vi "未命名 3.vi"(0 "Image In":T3, 1 "Image Dst":T3, 2 "ROI Descriptor (Pattern Matching 1)":T2={"Global Rectangle"=[20, 78, 890, 919], "Contours"=[{"ID"=enum."External", "Type"=12, "Coordinates"=[20, 78, 890, 919, 0]}]} {"Contours"."Type" items=["No Selection", "Point", "Line", "Rectangle", "Oval", "Polygon", "Freehand Region", "Annulus", "Unused2", "Unused3", "Broken Line", "Freehand Line", "Rotated Rectangle"]}, 3 "Algorithm (Pattern Matching 1)":i32(ring)=2 items=["All", "Low Discrepancy Sampling", "Grayscale Value Pyramid", "Gradients Pyramid"], 4 "Parameters (Pattern Matching 1)":T1={"Number of Matches Requested"=1, "Minimum Match Score"=800.0, "Angle Ranges"=[]}, 5 "Advanced Options (Pattern Matching 1)":cluster{"Item":u16, "Value":dbl}[](array[cluster])=[{"Item"=102, "Value"=10.0}, {"Item"=106, "Value"=300.0}, {"Item"=107, "Value"=0.0}, {"Item"=108, "Value"=6.0}, {"Item"=109, "Value"=1.0}, {"Item"=114, "Value"=25.0}, {"Item"=111, "Value"=20.0}, {"Item"=112, "Value"=10.0}, {"Item"=113, "Value"=20.0}, {"Item"=103, "Value"=1.0}, {"Item"=104, "Value"=20.0}, {"Item"=105, "Value"=0.0}, {"Item"=100, "Value"=6.0}] {"Item" items=["LD Sampling - Minimum Constrast"=0, "LD Sampling - Enable Subpixel Accuracy"=1, "LD Sampling - Search Strategy"=2, "LD Sampling - Subpixel Iterations"=3, "LD Sampling - Subpixel Tolerance"=4, "LD Sampling - Initial Match List Length"=5, "LD Sampling - Match List Reduction Factor"=6, "LD Sampling - Initial Step Size"=7, "LD Sampling - Intermediate Angular Accuracy"=8, "-"=9, "Pyramid - Max Pyramid Level"=100, "Pyramid - Minimum Contrast"=102, "Pyramid - Enable Subpixel Accuracy"=103, "Pyramid - Subpixel Iterations"=104, "Pyramid - Subpixel Tolerance"=105, "Pyramid - Initial Match List Length"=106, "Pyramid - Match List Reduction Factor"=107, "Pyramid - Intermediate Angular Accuracy"=108, "Pyramid - Process Border Matches"=109, "Pyramid - Min Match Separation Distance"=111, "Pyramid - Min Match Separation Angle"=112, "Pyramid - Max Match Overlap"=113, "Pyramid - Max Cache in MB"=114, "Pyramid - Clear Cache"=115, "-"=116, "Enable Defect Map"=200]}, 6 "Template File Path (Pattern Matching 1)":path=path "D:/Inspect System/Source Code/Template Program/字符检测定位模板.png", 7 "error in":errorcluster) -> (20 "Image Out":T3, 21 "Matches (Pattern Matching 1)":T4(array[cluster]) {"Bounding Box"."y" format="%.2f"; "Bounding Box"."x" format="%.2f"; "Position"."y" format="%.2f"; "Position"."x" format="%.2f"; "Score" format="%.2f"; "Scale" format="%.2f"; "Angle" format="%.2f"}, 22 "Calibrated Matches (Pattern Matching 1)":T4(array[cluster]) {"Bounding Box"."y" format="%.2f"; "Bounding Box"."x" format="%.2f"; "Position"."y" format="%.2f"; "Position"."x" format="%.2f"; "Score" format="%.2f"; "Scale" format="%.2f"; "Angle" format="%.2f"}, 23 "Number of Matches (Pattern Matching 1)":i32, 27 "error out":errorcluster)   [LabVIEW 2017]
doc: "Creates, edits, and runs vision algorithms using NI Vision Assistant.\n\nWhen you place this Express VI on the block diagram, NI Vision Assistant launches. Create an algorithm using the Vision Assistant processing functions. After you create an algorithm, you can select the controls and indicators that you want to be able to programmatically set in LabVIEW. Double-click the Vision Assistant Express VI to edit the algorithm."
uses:
  <vilib>/vision/Image Controls.llb/IMAQ Image.ctl
  <vilib>/vision/NI_Vision_Development_Module.lvlib
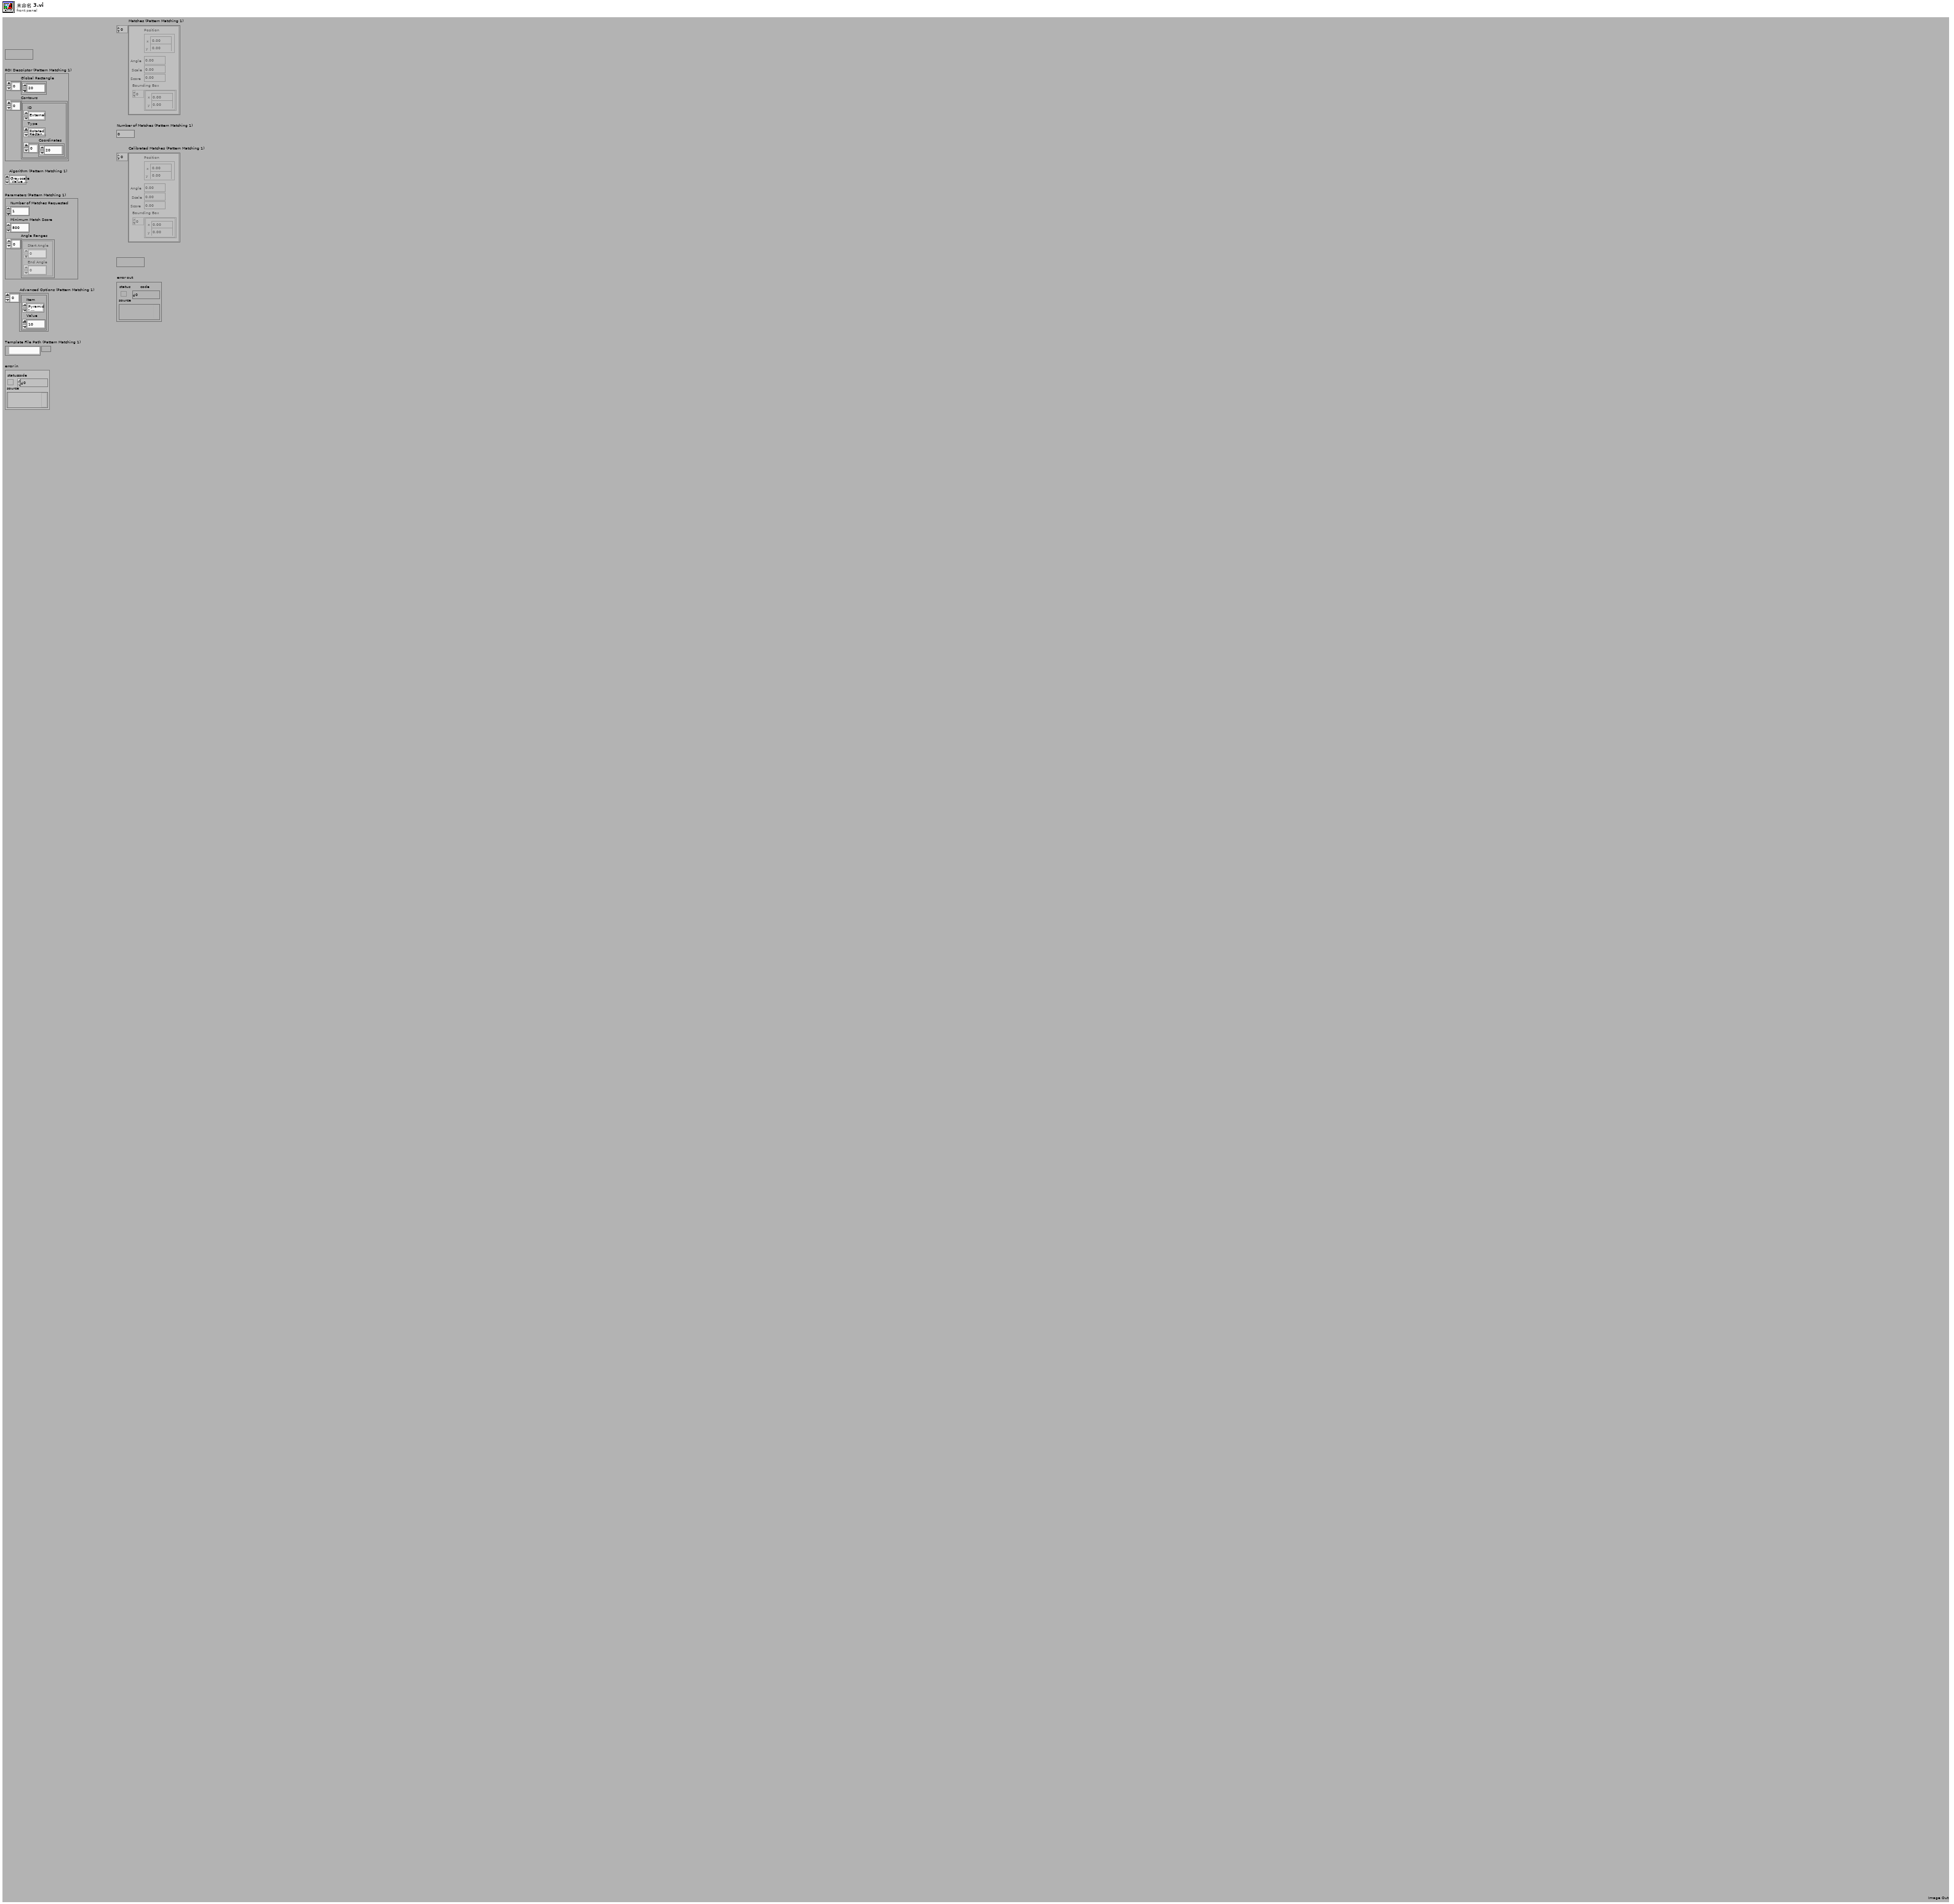
[diagram p1: front panel]
types:
  T1 = cluster{"Number of Matches Requested":i32, "Minimum Match Score":sgl, "Angle Ranges":cluster{"Start Angle":sgl, "End Angle":sgl}[]}
  T2 = cluster{"Global Rectangle":i32[], "Contours":cluster{"ID":enum32{"External", "Internal"}, "Type":u32, "Coordinates":i32[]}[]}
  T3 = typedef "IMAQ Image.ctl" = refnum<image>
  T4 = cluster{"Position":cluster{"x":sgl, "y":sgl}, "Angle":sgl, "Scale":sgl, "Score":sgl, "Bounding Box":cluster{"x":sgl, "y":sgl}[]}[]
  T5 = typedef "Image Type" = u32
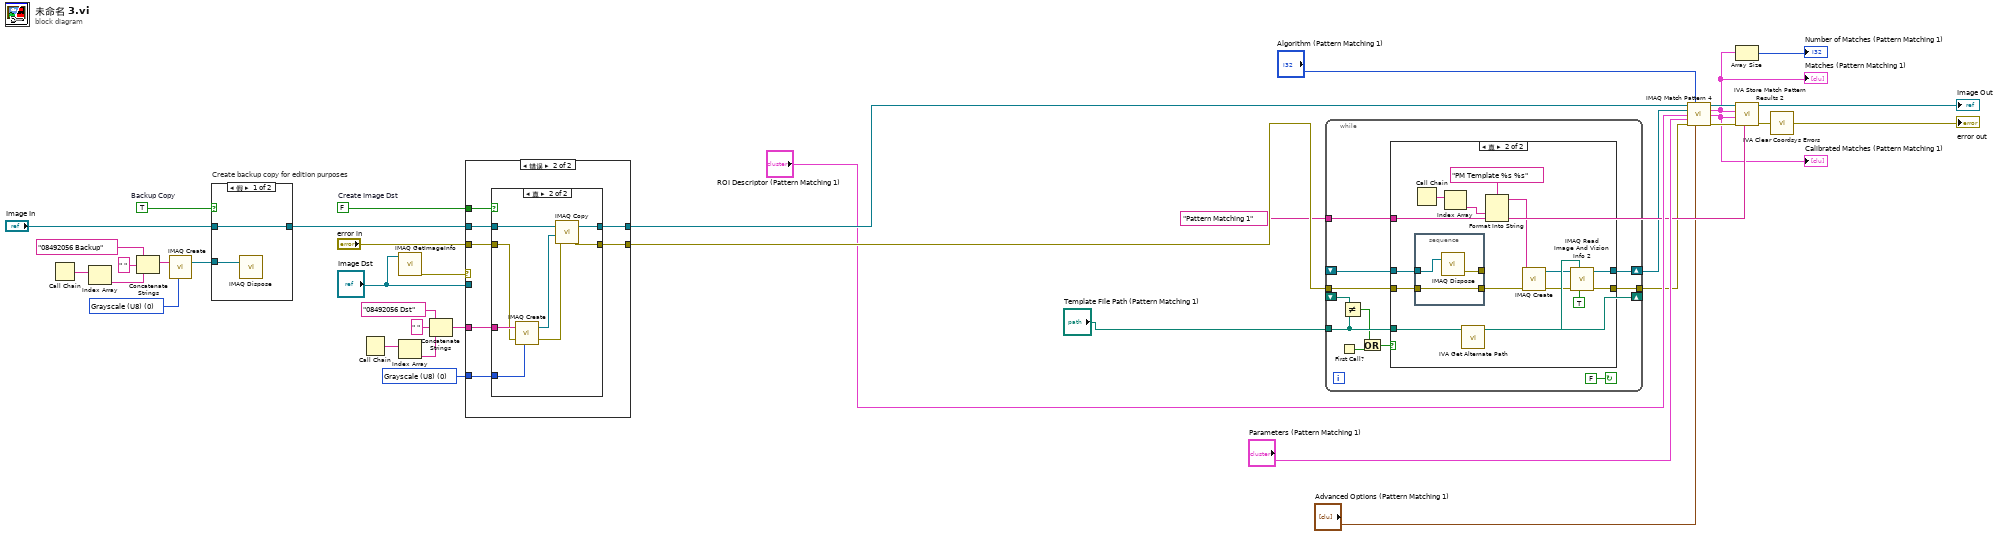
[diagram p0: block diagram]
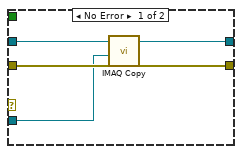
[diagram p3: hidden frame]
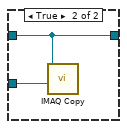
[diagram p5: hidden frame]
diagram:
  w9 = "Pattern Matching 1" ("Step Name")
  w18 = T5 0 items=["Grayscale (U8)", "Grayscale (I16)", "Grayscale (SGL)", "Complex (CSG)", "RGB (U32)", "HSL (U32)", "RGB (U64)", "Grayscale (U16)"] ("Image Dst Type")
  w19 = T5 0 items=["Grayscale (U8)", "Grayscale (I16)", "Grayscale (SGL)", "Complex (CSG)", "RGB (U32)", "HSL (U32)", "RGB (U64)", "Grayscale (U16)"] ("Image Type")
  w38 = TRUE  # Backup Copy
  w31 = FALSE  # Create Image Dst
  n1 = Call Chain() -> (call chain=w25:string[])
  n2 = Index Array(array=w25) -> (element=w24:string)  [unwired: 1 in]
  n3 = Concatenate Strings("08492056 Backup" ("Backup Image Name"), " ", w24) -> (w21:string)
  n4 = call "IMAQ Create"("Image Name"=w21, "Image Type"=w19) -> ("New Image"=w20:T3)  [unwired: 2 in, 2 out]
  n5 = case "Create backup copy for edition purposes" shown="假" w38 {
    tunnel: [w40 w42] -> w34
    tunnel: "Image In" -> [w40 w42]
    tunnel: w20 -> [w39 w41]
    frame False {
      n6 = call "IMAQ Dispose"("Image"=w39) -> ()  [unwired: 2 in, 4 out]
    }
    frame True {
      n7 = call "IMAQ Copy"("Image Dst"=w41, "Image Src"=w42) -> ()  [unwired: 1 in, 5 out]
    }
  }
  n8 = Call Chain() -> (call chain=w30:string[])
  n9 = call "IMAQ GetImageInfo"("Image"="Image Dst") -> ("error out"=w36:errorcluster)  [unwired: 1 in, 9 out]
  n10 = Index Array(array=w30) -> (element=w28:string)  [unwired: 1 in]
  n11 = Concatenate Strings("08492056 Dst" ("Image Dst Name"), " ", w28) -> (w26:string)
  n12 = case "条件结构" shown="错误" w36 {
    tunnel: [w47 w51] -> w16
    tunnel: [w46 w50] -> w32
    tunnel: w34 -> [w45 w52]
    tunnel: "error in" -> [w44 w48]
    tunnel: "Image Dst" -> [w43 _]
    tunnel: w26 -> [_ w54]
    tunnel: w18 -> [_ w53]
    tunnel: w31 -> [_ w49]
    frame No Error {
      n13 = call "IMAQ Copy"("error in (no error)"=w44, "Image Dst"=w43, "Image Src"=w45) -> ("error out"=w46:errorcluster, "Image Dst Out"=w47:T3)  [unwired: 3 out]
    }
    frame Error {
      n14 = case "条件结构" shown="真" w49 {
        tunnel: w54 -> [_ w64]
        tunnel: w53 -> [_ w63]
        tunnel: w52 -> [w56 w61]
        tunnel: [w56 w60] -> w51
        tunnel: [w55 w59] -> w50
        tunnel: w48 -> [w55 w57]
        frame False {
        }
        frame True {
          n15 = call "IMAQ Create"("Image Name"=w64, "Image Type"=w63, "error in (no error)"=w57) -> ("New Image"=w62:T3, "error out"=w58:errorcluster)  [unwired: 1 in, 1 out]
          n16 = call "IMAQ Copy"("error in (no error)"=w58, "Image Dst"=w62, "Image Src"=w61) -> ("error out"=w59:errorcluster, "Image Dst Out"=w60:T3)  [unwired: 3 out]
        }
      }
    }
  }
  n17 = while {
    shift-right: [w75] -> w6
    shift-left: _ -> [w74]
    tunnel: [w72] -> w5
    tunnel: w32 -> [w71]
    tunnel: "Template File Path (Pattern Matching 1)" -> [w68]
    tunnel: w9 -> [w70]
    shift-right: [w68] -> _
    shift-left: _ -> [w69]
    stop <- FALSE continue-if-true
    n18 = First Call?() -> (First Call?: T/F=w67:bool)
    n19 = Not Equal?(x=w69, y=w68) -> (x != y?=w66:bool)
    n20 = Or(x=w66, y=w67) -> (x .or. y?=w65:bool)
    n21 = case "条件结构" shown="真" w65 {
      tunnel: [w77 w82] -> w75
      tunnel: w74 -> [w77 w86]
      tunnel: [w76 w83] -> w72
      tunnel: w71 -> [w76 w85]
      tunnel: w68 -> [_ w87]
      tunnel: w70 -> [_ w88]
      frame False {
      }
      frame True {
        n22 = stacked-sequence "层叠式顺序结构" {
          tunnel: w86 -> [w95]
          tunnel: w85 -> [w94]
          tunnel: [w94] -> w79
          tunnel: [w93] -> _
          frame #0 {
            n23 = call "IMAQ Dispose"("Image"=w95) -> ("error out"=w93:errorcluster)  [unwired: 2 in, 3 out]
          }
        }
        n24 = Call Chain() -> (call chain=w90:string[])
        n25 = Index Array(array=w90) -> (element=w89:string)  [unwired: 1 in]
        n26 = call <vilib>:"IVA Get Alternate Path.vi"("Path In"=w87) -> ("Path Out"=w84:path)  [unwired: 10 out]
        n27 = Format Into String(format string="PM Template %s %s" ("Image Name"), w89, w88) -> (resulting string=w92:string)  [unwired: 2 in, 1 out]
        n28 = call "IMAQ Create"("Image Name"=w92, "error in (no error)"=w79) -> ("New Image"=w81:T3, "error out"=w80:errorcluster)  [unwired: 2 in, 1 out]
        n29 = call "IMAQ Read Image And Vision Info 2"("Use File Path Image Type"=TRUE, "File Path"=w84, "error in (no error)"=w80, "Image"=w81) -> ("error out"=w83:errorcluster, "Image Out"=w82:T3)  [unwired: 5 in, 1 out]
      }
    }
  }
  n30 = call "IMAQ Match Pattern 4"("Image"=w16, "Algorithm"="Algorithm (Pattern Matching 1)", "Template Image"=w6, "ROI Descriptor"="ROI Descriptor (Pattern Matching 1)", "Parameters"="Parameters (Pattern Matching 1)", "error in (no error)"=w5, "Advanced Options"="Advanced Options (Pattern Matching 1)") -> ("Image (duplicate)"=w14:T3, "Matches (pixel)"=w8:T4, "Matches (real-world)"=w7:T4, "error out"=w15:errorcluster)  [unwired: 4 in, 1 out]
  "Matches (Pattern Matching 1)" <- w8
  "Calibrated Matches (Pattern Matching 1)" <- w7
  n31 = Array Size(array=w8) -> (size(s)=→"Number of Matches (Pattern Matching 1)":i32)
  n32 = call <vilib>:"IVA Store Match Pattern Results 2.vi"("Step Name"=w9, "error in (no error)"=w15, "Matches (real-world)"=w7, "Matches (pixel)"=w8, "Image in"=w14) -> ("error out"=w4:errorcluster, "Image dup"=→"Image Out":T3)  [unwired: 1 in, 4 out]
  n33 = call <vilib>:"IVA Clear Coordsys Errors.vi"("error in (no error)"=w4) -> ("error out"=→"error out":errorcluster)  [unwired: 10 in]
